vi "Get Frame Metadata Size.vi"(10 "pMetadataSize":i32, 11 "index":u16) -> (2 "pMetadataSize out":i32, 3 "function return":i32)   [LabVIEW 2025, in "ExtremelyEpicImagerIPC2.lvlib"]
doc: "IMAGERIPC_API HRESULT WINAPI GetFrame(WORD index, WORD timeout, void *pBuf, unsigned int Size, FrameMetadata *pMetadata); IMAGERIPC_API HRESULT WINAPI GetVisibleFrame(WORD index, WORD timeout, void *pBuf, unsigned int Size, FrameMetadata *pMetadata); IMAGERIPC_API HRESULT WINAPI GetFrameMetadataSize(WORD index, int *pMetadataSize);"
uses:
  ExtremelyEpicImagerIPC2.lvlib
  ImagerIPC2.dll
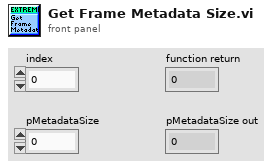
[diagram p1: front panel]
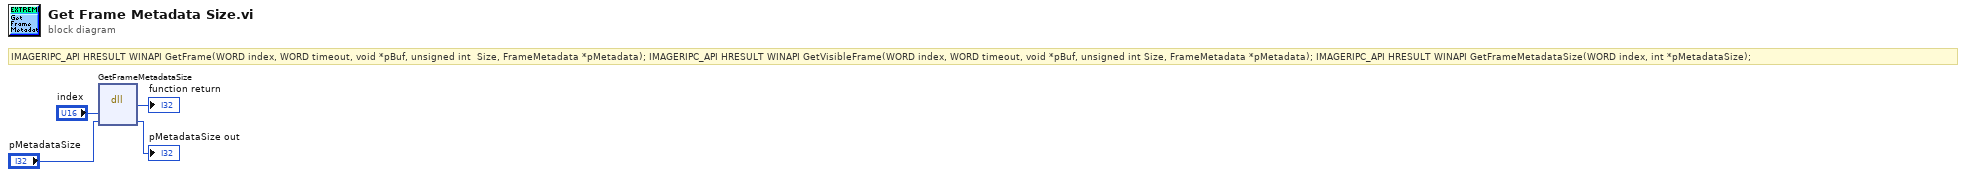
[diagram p0: block diagram]
diagram:
  # "IMAGERIPC_API HRESULT WINAPI GetFrame(WORD index, WORD timeout, void *pBuf, unsigned int  Size, FrameMetadata *pMetadata); IMAGERIPC_API HRESULT WINAPI GetVisibleFrame(WORD index, WORD timeout, void *pBuf, unsigned int Size, FrameMetadata *pMetadata); IMAGERIPC_API HRESULT WINAPI GetFrameMetadataSize(WORD index, int *pMetadataSize);"
  n1 = dll-call lib="C:/Users/mayhe/OneDrive/Documents/GitHub/In-situ-monitoring-of-powder-bed-fusion-additive-manufacturing/system_development/Orichalcum/v0.2/Software_design/thermal-camera/VI/Connect SDK/ImagerIPC2.*" fn="GetFrameMetadataSize"("index"="index", "pMetadataSize"="pMetadataSize") -> (→"function return":i32, "pMetadataSize"=→"pMetadataSize out":i32)  [unwired: 4 in, 2 out]
